vi "CE Calculate Fit.vi"(8 "error in (no error)":errorcluster, 10 "CE measurement":T2={"Signal frequencies (Hz) T"=[1000.0], "Signal amplitudes (V) T"=[0.707], "Sampling frequencies (Hz) T"=[10000000.0], "Record lengths (multiples of periods) T"=[10000.0], "TWM data root directory"=path "", "TWM mreasurements directories"=[], "Calculate RMS from samples"=FALSE, "Algorithm to use"="TWM-WFFT", "Quantity to read"="TWM-WFFT", "Settle down after AC source change (s) T"=1.0, "Skip PJVS setup"=FALSE, "Measurement template file"=path "", "Row of START keyword T"=0, "Row of STOP keyword T"=0, "Measurement template line T"=[], "Switch position T"=[10000.0], "FR fit mat file T"=path "", "Recalculate-skip already calculated"=FALSE} {"Switch position T" format="%#_3p"; "Record lengths (multiples of periods) T" format="%#_3p"; "Sampling frequencies (Hz) T" format="%#_3p"; "Signal amplitudes (V) T" format="%#_3p"; "Signal frequencies (Hz) T" format="%#_3p"}, 11 "Common properties":T1={"Measurement status ref"=refnum, "TWM Status ref"=refnum, "Abort ref"=refnum, "Skip waiting ref"=refnum, "GNU Octave path"=path "C:/Program Files/GNU Octave/Octave-6.2.0/mingw64/bin", "TWM+QWTB path"=path "C:/Users/labina/Desktop/TWM-1.8.7.0-full/octprog", "lvlib path"=path "D:/martin/WAC/WACsw - github/control_software/Filter function meter/external libraries/GOLPI 0.7.3.1 source distribution LV 20.0 32 bit/lv_proc.dll", "TWM pipe"="\\\\.\\pipe\\TWM:server", "PJVS status ref"=refnum, "WAC path"=path ""}) -> (0 "error out":errorcluster)   [LabVIEW 2020]
doc: "Runs calculation of CE measurement using read_M_CE_from_spreadsheet.m and P_CE.m scripts."
uses:
  CE Measurement/Type definitions/CE measurement.ctl
  Utilities/Type definitions/Common properties.ctl
  Utilities/Calculation related/Globals for GOLPI.vi
  external libraries/GOLPI 0.7.3.1 source distribution LV 20.0 32 bit/GOLPI library.lvlib
panel:
  out "command\n(for debug)":string="addpath('info'); addpath('qwtb'); qwtb_exec_algorithm('%s', 0, 1); disp('FINISHEDCR')"
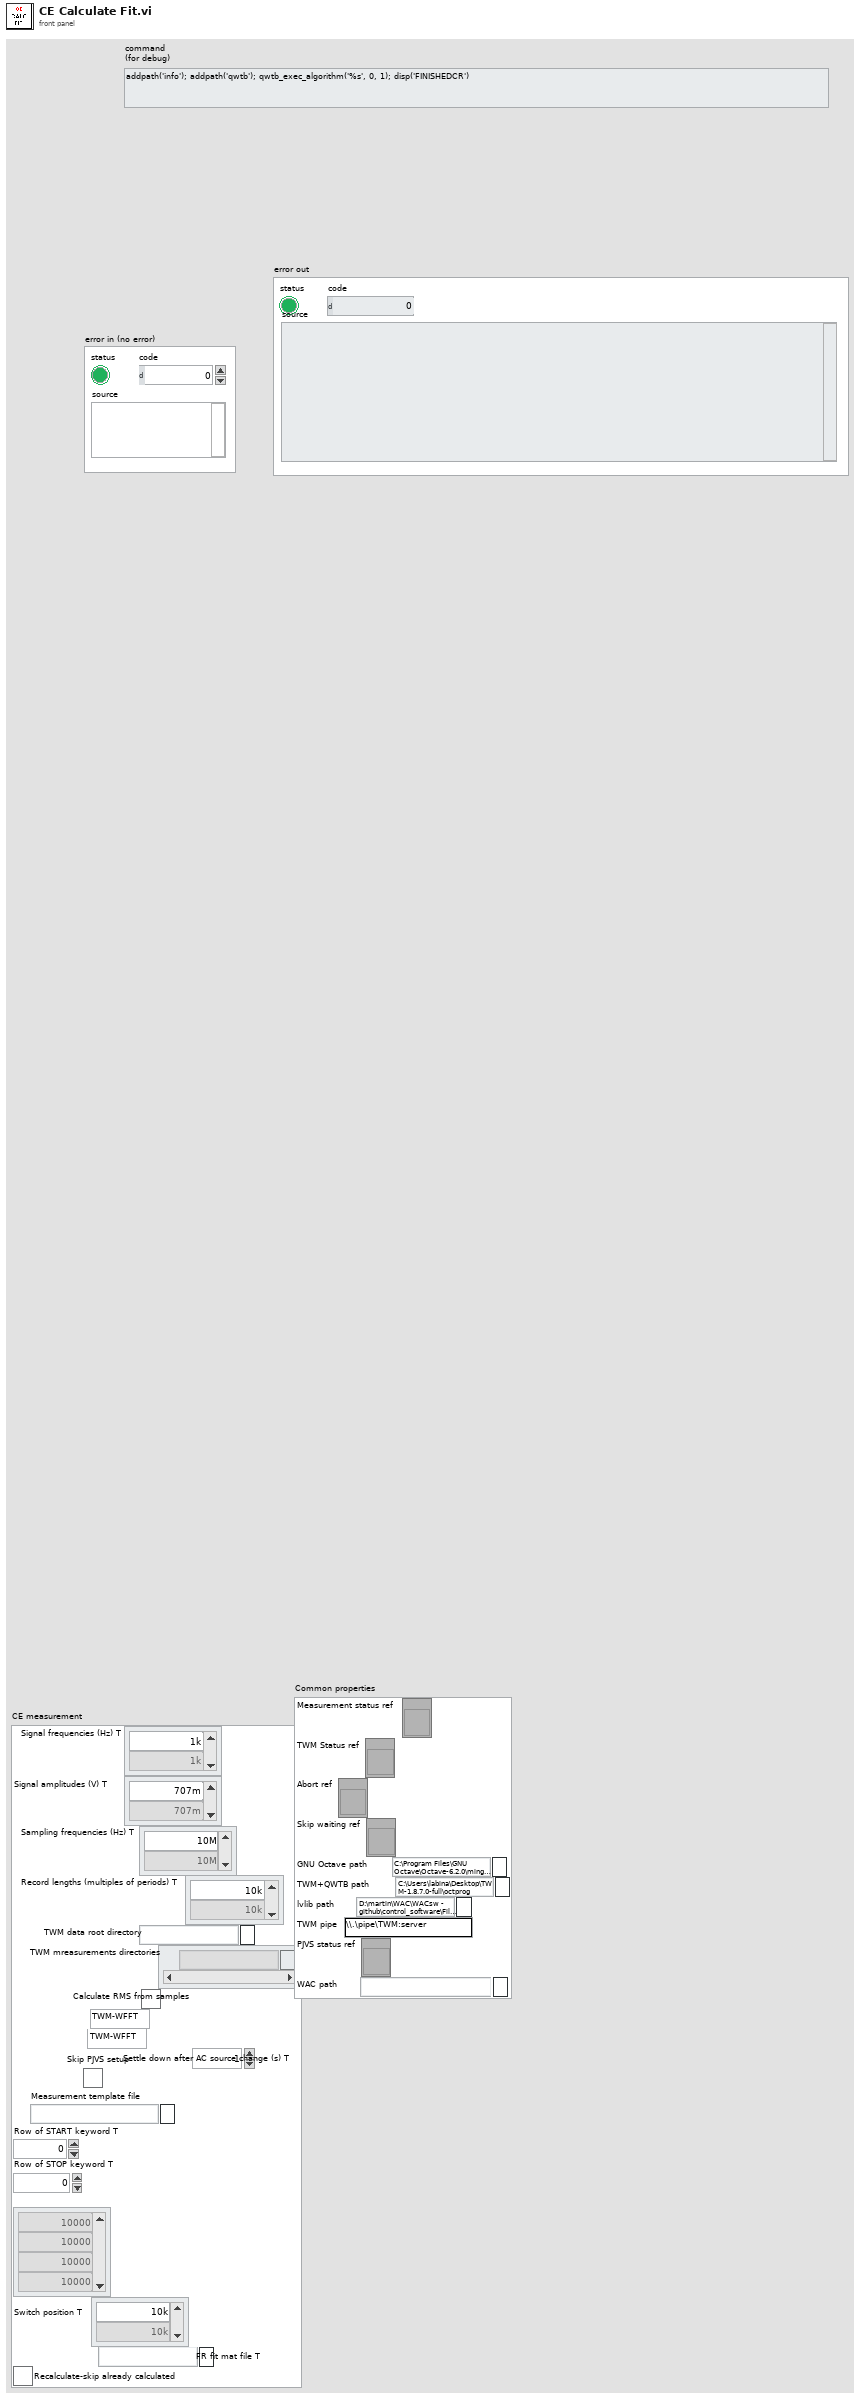
[diagram p1: front panel]
types:
  T1 = typedef "Common properties.ctl" = cluster{"Measurement status ref":refnum<vi>, "TWM Status ref":refnum<vi>, "Abort ref":refnum<vi>, "Skip waiting ref":refnum<vi>, "GNU Octave path":path, "TWM+QWTB path":path, "lvlib path":path, "TWM pipe":string, "PJVS status ref":refnum<vi>, "WAC path":path}
  T2 = typedef "CE measurement.ctl" = cluster{"Signal frequencies (Hz) T":dbl[], "Signal amplitudes (V) T":dbl[], "Sampling frequencies (Hz) T":dbl[], "Record lengths (multiples of periods) T":dbl[], "TWM data root directory":path, "TWM mreasurements directories":path[], "Calculate RMS from samples":bool, "Algorithm to use":string, "Quantity to read":string, "Settle down after AC source change (s) T":dbl, "Skip PJVS setup":bool, "Measurement template file":path, "Row of START keyword T":i32, "Row of STOP keyword T":i32, "Measurement template line T":i32[], "Switch position T":dbl[], "FR fit mat file T":path, "Recalculate-skip already calculated":bool}
  T3 = typedef "GOLPI library.lvlib/GOLPI reference Type Def.ctl" = cluster{"pipe handle":T4, "fast read timeout [ms]":u32, "fast read settle time [ms]":u32, "fast read to multiple [ms]":u32, "max elements per input line":u32, "slow read timeout [ms]":u32, "stdin double format specifier":string, "max elements per stdout output column":u32, "console mode bitstream":bool, "bitstream first read timeout [ms]":u32, "bitstream read timeout [ms]":u32, "struct transfer possible":bool, "matlab mode":bool}
  T4 = typedef "LV Process library.lvlib/Pipe Handle.ctl" = cluster{"lv_proc.dll file path":path, "process instance handle":u32[], "debug mode":bool, "debug data":cluster{"time":timestamp, "stdin":bool, "data":string}[]}
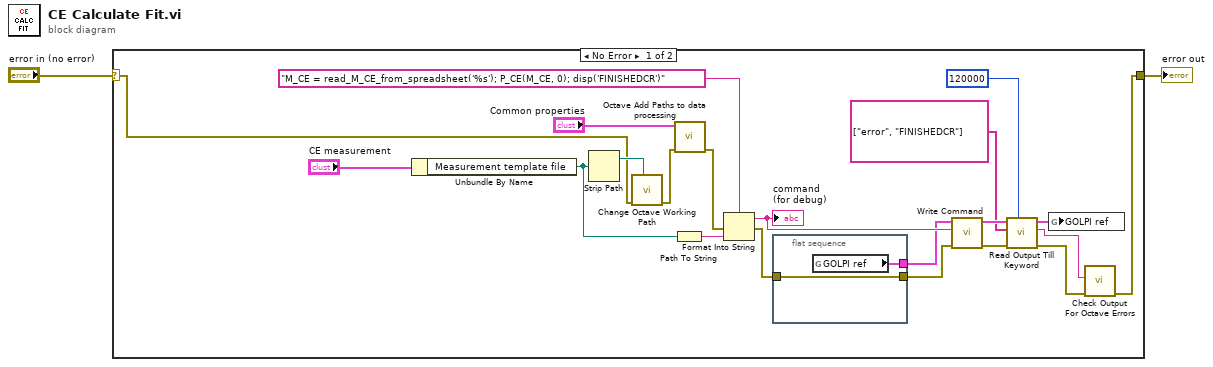
[diagram p0: block diagram]
diagram:
  n1 = case shown="No Error" "error in (no error)" {
    selector: "error in (no error)" -> [w14 w26]
    tunnel: [w4 w26] -> w2
    frame No Error {
      n2 = Unbundle By Name("CE measurement") -> ("Measurement template file"=w13:path)
      n3 = Strip Path(path=w13) -> (stripped path=w16:path)  [unwired: 1 out]
      n4 = call "Change Octave Working Path.vi"("Measurement path in"=w16, "error in (no error)"=w14) -> ("error out"=w8:errorcluster)  [unwired: 9 in]
      n5 = Path To String(path=w13) -> (string=w22:string)
      n6 = call "Octave Add Paths to data processing.vi"("error in (no error)"=w8, "Common properties"="Common properties") -> ("error out"=w7:errorcluster)  [unwired: 9 in]
      n7 = Format Into String(format string="M_CE = read_M_CE_from_spreadsheet('%s'); P_CE(M_CE, 0); disp('FINISHEDCR')", error in=w7, w22) -> (resulting string=w17:string, error out=w12:errorcluster)  [unwired: 1 in]
      "command\n(for debug)" <- w17
      n8 = flat-sequence {
        tunnel: [w25] -> w11
        tunnel: w12 -> [w25]
        tunnel: [w24] -> w10
        frame #0 {
          n9 = global read "Globals for GOLPI.vi" "GOLPI ref"() -> (w24:T3)
        }
      }
      n10 = call "Write Command.vi"("error in"=w11, "command"=w17, "GOLPI ref. in"=w10) -> ("error out"=w21:errorcluster, "GOLPI ref. out"=w20:T3)  [unwired: 7 in]
      n11 = call "Read Output Till Keyword.vi"("timeout [ms]"=u32 120000, "error in"=w21, "keywords"=string[] ["error", "FINISHEDCR"], "GOLPI ref. in"=w20) -> ("error out"=w5:errorcluster, "read buffer"=w3:string, "GOLPI ref. out"=w9:T3)  [unwired: 4 in, 1 out]
      n12 = global write "Globals for GOLPI.vi" "GOLPI ref"(w9) -> ()
      n13 = call "Check Output For Octave Errors.vi"("error in"=w5, "read buffer"=w3) -> ("error out"=w4:errorcluster)  [unwired: 9 in]
    }
    frame Error {
    }
  }
  "error out" <- w2
